vi "Register HVAC System View.vi"(11 "Message Enqueuer in":refnum<class "Message Enqueuer.lvclass">) -> (3 "Message Enqueuer out":refnum<class "Message Enqueuer.lvclass">)   [LabVIEW 2013]
uses:
  <vilib>/ActorFramework/Message Enqueuer/Message Enqueuer.lvclass
  <vilib>/ActorFrameworkMVC/View Observer/Registration Message/Registration Message.lvclass
  <vilib>/ActorFrameworkMVC/View Observer/Data Message/Data Message.lvclass
  Models/HVAC System Model Messages/Register HVAC System Move In Next Msg/Register HVAC System Move In Next Msg.lvclass
  Models/HVAC System Model Messages/Register HVAC System Move In Previous Msg/Register HVAC System Move In Previous Msg.lvclass
  Models/HVAC System Model Messages/Register HVAC System Next Button Visibility Msg/Register HVAC System Next Button Visibility Msg.lvclass
  Models/HVAC System Model Messages/Register HVAC System Previous Button Visibility Msg/Register HVAC System Previous Button Visibility Msg.lvclass
  Models/HVAC System Model Messages/Register HVAC System Tiles Info Msg/Register HVAC System Tiles Info Msg.lvclass
  Views/HVAC System View Messages/Conceret HVAC System Move In Next Msg/Conceret HVAC System Move In Next Msg.lvclass
  Views/HVAC System View Messages/Conceret HVAC System Move In Previous Msg/Conceret HVAC System Move In Previous Msg.lvclass
  Views/HVAC System View Messages/Conceret HVAC System Next Button Visibility Msg/Conceret HVAC System Next Button Visibility Msg.lvclass
  Views/HVAC System View Messages/Conceret HVAC System Previous Button Visibility Msg/Conceret HVAC System Previous Button Visibility Msg.lvclass
  Views/HVAC System View Messages/Conceret HVAC System Tiles Info Msg/Conceret HVAC System Tiles Info Msg.lvclass
  <vilib>/ActorFrameworkMVC/UI Controller Messages/Subscribe View to Model Msg/Subscribe View to Model Msg.lvclass/Subscribe View to Model Msg.ctl
  <vilib>/ActorFramework/Message Enqueuer/Message Enqueuer.lvclass/Message Enqueuer.ctl
  <vilib>/ActorFramework/Message Enqueuer/Enqueue.vi
  <vilib>/ActorFramework/Message Priority Queue/Priority Enqueue.vi
  <vilib>/ActorFrameworkMVC/UI Controller Messages/Subscribe View to Model Msg/Subscribe View to Model Msg.lvclass
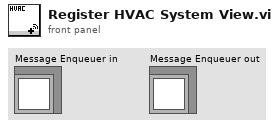
[diagram p1: front panel]
types:
  T1 = cluster{"Registration Message":string, "Data Message":string}[]
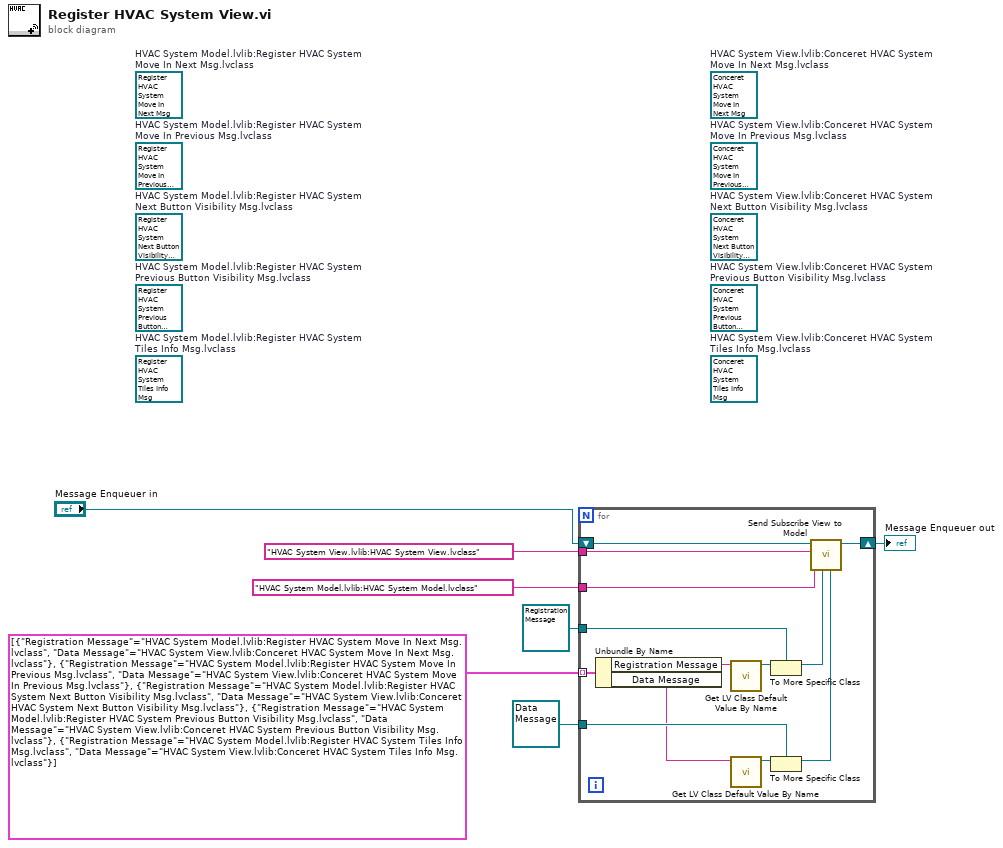
[diagram p0: block diagram]
diagram:
  (unwired) refnum<class "Conceret HVAC System Tiles Info Msg.lvclass"> refnum  # HVAC System View.lvlib:Conceret HVAC System Tiles Info Msg.lvclass
  (unwired) refnum<class "Conceret HVAC System Previous Button Visibility Msg.lvclass"> refnum  # HVAC System View.lvlib:Conceret HVAC System Previous Button Visibility Msg.lvclass
  (unwired) refnum<class "Conceret HVAC System Next Button Visibility Msg.lvclass"> refnum  # HVAC System View.lvlib:Conceret HVAC System Next Button Visibility Msg.lvclass
  (unwired) refnum<class "Conceret HVAC System Move In Previous Msg.lvclass"> refnum  # HVAC System View.lvlib:Conceret HVAC System Move In Previous Msg.lvclass
  (unwired) refnum<class "Conceret HVAC System Move In Next Msg.lvclass"> refnum  # HVAC System View.lvlib:Conceret HVAC System Move In Next Msg.lvclass
  (unwired) refnum<class "Register HVAC System Tiles Info Msg.lvclass"> refnum  # HVAC System Model.lvlib:Register HVAC System Tiles Info Msg.lvclass
  (unwired) refnum<class "Register HVAC System Previous Button Visibility Msg.lvclass"> refnum  # HVAC System Model.lvlib:Register HVAC System Previous Button Visibility Msg.lvclass
  (unwired) refnum<class "Register HVAC System Next Button Visibility Msg.lvclass"> refnum  # HVAC System Model.lvlib:Register HVAC System Next Button Visibility Msg.lvclass
  (unwired) refnum<class "Register HVAC System Move In Previous Msg.lvclass"> refnum  # HVAC System Model.lvlib:Register HVAC System Move In Previous Msg.lvclass
  (unwired) refnum<class "Register HVAC System Move In Next Msg.lvclass"> refnum  # HVAC System Model.lvlib:Register HVAC System Move In Next Msg.lvclass
  n1 = for {
    tunnel: "HVAC System View.lvlib:HVAC System View.lvclass" ("View Name") -> [w19]
    tunnel: "HVAC System Model.lvlib:HVAC System Model.lvclass" ("Model Name") -> [w18]
    shift-right: [w17] -> w7
    shift-left: "Message Enqueuer in" -> [w20]
    tunnel: refnum<class "Registration Message.lvclass"> refnum ("Registration Message") -> [w14]
    tunnel: refnum<class "Data Message.lvclass"> refnum ("Data Message") -> [w13]
    tunnel: T1 [{"Registration Message"="HVAC System Model.lvlib:Register HVAC System Move In Next Msg.lvclass", "Data Message"="HVAC System View.lvlib:Conceret HVAC System Move In Next Msg.lvclass"}, {"Registration Message"="HVAC System Model.lvlib:Register HVAC System Move In Previous Msg.lvclass", "Data Message"="HVAC System View.lvlib:Conceret HVAC System Move In Previous Msg.lvclass"}, {"Registration Message"="HVAC System Model.lvlib:Register HVAC System Next Button Visibility Msg.lvclass", "Data Message"="HVAC System View.lvlib:Conceret HVAC System Next Button Visibility Msg.lvclass"}, {"Registration Message"="HVAC System Model.lvlib:Register HVAC System Previous Button Visibility Msg.lvclass", "Data Message"="HVAC System View.lvlib:Conceret HVAC System Previous Button Visibility Msg.lvclass"}, {"Registration Message"="HVAC System Model.lvlib:Register HVAC System Tiles Info Msg.lvclass", "Data Message"="HVAC System View.lvlib:Conceret HVAC System Tiles Info Msg.lvclass"}] -> [w12] mode=indexing
    n2 = Unbundle By Name(w12) -> ("Registration Message"=w9:string, "Data Message"=w8:string)
    n3 = call <vilib>:"Get LV Class Default Value By Name.vi"("class name"=w9) -> ("object"=w16:refnum<class>)  [unwired: 9 in, 1 out]
    n4 = call <vilib>:"Get LV Class Default Value By Name.vi"("class name"=w8) -> ("object"=w15:refnum<class>)  [unwired: 9 in, 1 out]
    n5 = To More Specific Class(target class=w14, reference=w16) -> (specific class reference=w11:refnum<class "Registration Message.lvclass">)  [unwired: 1 in, 1 out]
    n6 = To More Specific Class(target class=w13, reference=w15) -> (specific class reference=w10:refnum<class "Data Message.lvclass">)  [unwired: 1 in, 1 out]
    n7 = call <vilib>:"Send Subscribe View to Model.vi"("Data Message"=w10, "Registration Message"=w11, "Model Name"=w18, "View Name"=w19, "Message Enqueuer"=w20) -> ("Message Enqueuer out"=w17:refnum<class "Message Enqueuer.lvclass">)  [unwired: 5 in, 1 out]
  }
  "Message Enqueuer out" <- w7
